vi "PCTime_to_GPSTime.vi"(2 "GPS time difference":i32, 3 "Current PC time":timestamp) -> (0 "GPS date/time string":string, 1 "Current GPS time":timestamp)   [LabVIEW 2012]
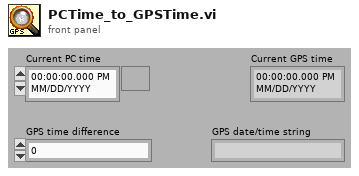
[diagram p1: front panel]
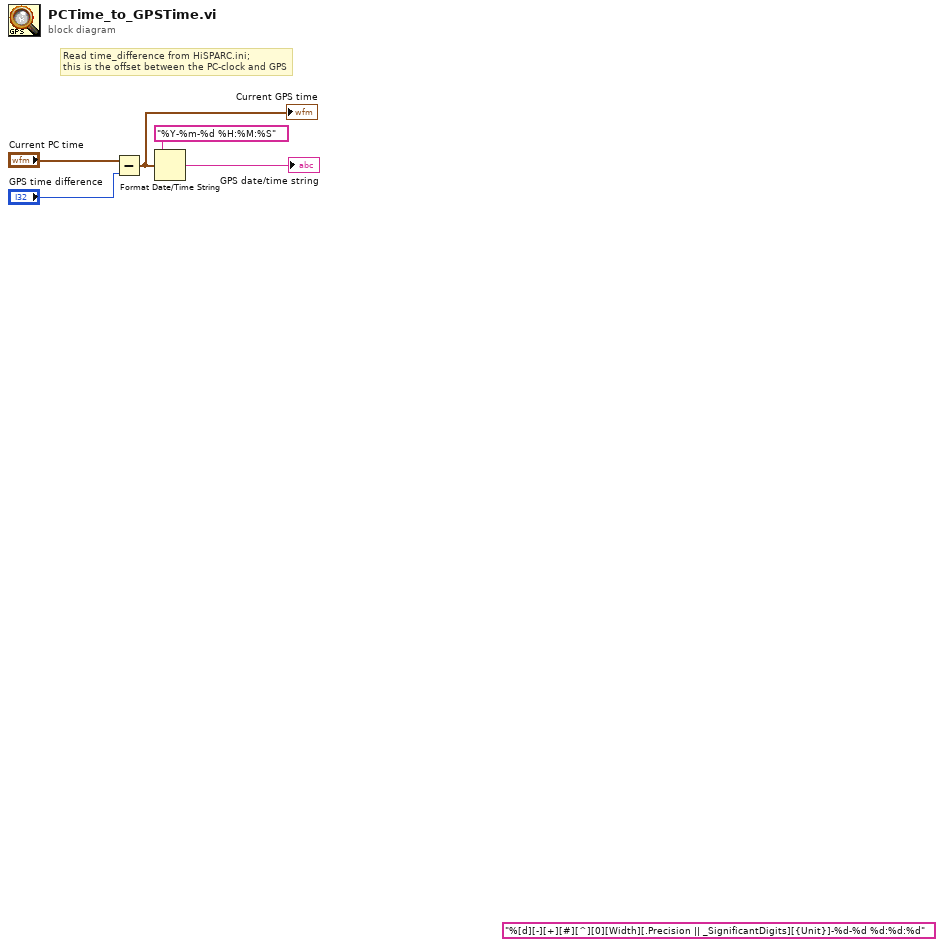
[diagram p0: block diagram]
diagram:
  (unwired) "%[d][-][+][#][^][0][Width][.Precision || _SignificantDigits][{Unit}]-%d-%d %d:%d:%d" ("format string")
  # "Read time_difference from HiSPARC.ini;\nthis is the offset between the PC-clock and GPS"
  n1 = Subtract(x="Current PC time", y="GPS time difference") -> (x-y=w2:timestamp)
  "Current GPS time" <- w2
  n2 = Format Date/Time String(time format string (%c)="%Y-%m-%d %H:%M:%S", seconds (now)=w2) -> (date/time string=→"GPS date/time string":string)  [unwired: 1 out]
